vi "toggle two.vi"(11 "Button In":bool) -> (3 "tggle Out":bool)   [LabVIEW 2012]
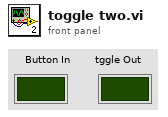
[diagram p1: front panel]
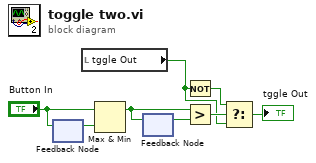
[diagram p0: block diagram]
diagram:
  n1 = feedback #1() -> (w6:bool)  [unwired: 1 in]
  n2 = feedback-in #1("Button In") -> ()
  n3 = local read "tggle Out"() -> (w1:bool)
  n4 = Max & Min(x="Button In", y=w6) -> (max(x,y)=w5:bool)  [unwired: 1 out]
  n5 = feedback #2() -> (w8:bool)  [unwired: 1 in]
  n6 = feedback-in #2(w5) -> ()
  n7 = Not(x=w1) -> (.not. x?=w2:bool)
  n8 = Greater?(x=w5, y=w8) -> (0:w4:bool)
  n9 = Select(t=w2, s=w4, f=w1) -> (s? t:f=→"tggle Out":bool)
